vi "SRV_Watchdog Check Time.vi"(0 "System Config":T1={"SRV IP Address"="", "Video Stream Rate Period (ms)"=250, "Enable Diagnostic Log"=FALSE, "Watchdog 1 Config"={"Watchdog Name"="", "Watchdog Period (s)"=1.0, "Watchdog Command"={"I2C Address"=0, "Register"=0, "Value"=0, "Active"=FALSE}}, "Watchdog 2 Config"={"Watchdog Name"="", "Watchdog Period (s)"=1.0, "Watchdog Command"={"I2C Address"=0, "Register"=0, "Value"=0, "Active"=FALSE}}, "Sensor Window Filepath"=path ""} {"Watchdog 2 Config"."Watchdog Period (s)" format="%.3f"; "Watchdog 2 Config"."Watchdog Command"."Value" format="%02x"; "Watchdog 2 Config"."Watchdog Command"."Register" format="%02x"; "Watchdog 2 Config"."Watchdog Command"."I2C Address" format="%02x"; "Watchdog 1 Config"."Watchdog Period (s)" format="%.3f"; "Watchdog 1 Config"."Watchdog Command"."Value" format="%02x"; "Watchdog 1 Config"."Watchdog Command"."Register" format="%02x"; "Watchdog 1 Config"."Watchdog Command"."I2C Address" format="%02x"}, 7 "WD 1 Last Update":dbl, 9 "WD 2 Last Update":dbl, 11 "error in (no error)":errorcluster) -> (4 "System Config dup":T1={"SRV IP Address"="", "Video Stream Rate Period (ms)"=250, "Enable Diagnostic Log"=FALSE, "Watchdog 1 Config"={"Watchdog Name"="", "Watchdog Period (s)"=1.0, "Watchdog Command"={"I2C Address"=0, "Register"=0, "Value"=0, "Active"=FALSE}}, "Watchdog 2 Config"={"Watchdog Name"="", "Watchdog Period (s)"=1.0, "Watchdog Command"={"I2C Address"=0, "Register"=0, "Value"=0, "Active"=FALSE}}, "Sensor Window Filepath"=path ""} {"Watchdog 2 Config"."Watchdog Period (s)" format="%.3f"; "Watchdog 2 Config"."Watchdog Command"."Value" format="%02x"; "Watchdog 2 Config"."Watchdog Command"."Register" format="%02x"; "Watchdog 2 Config"."Watchdog Command"."I2C Address" format="%02x"; "Watchdog 1 Config"."Watchdog Period (s)" format="%.3f"; "Watchdog 1 Config"."Watchdog Command"."Value" format="%02x"; "Watchdog 1 Config"."Watchdog Command"."Register" format="%02x"; "Watchdog 1 Config"."Watchdog Command"."I2C Address" format="%02x"}, 6 "Current Time":dbl, 8 "Update WD 1?":bool, 10 "Update WD 2?":bool, 15 "error out":errorcluster)   [LabVIEW 2014]
uses:
  SubVIs/SysConfig/SRV_System Config.ctl
  SRV_Watchdog Config Cluster.ctl
  Motors/Motors Config/SRV_Motor Control Command Config.ctl
panel:
  # "I2C Address"
  # "Register"
  # "Value"
  # "Active"
  # "I2C Address"
  # "Register"
  # "Value"
  # "Active"
  # "I2C Address"
  # "Register"
  # "Value"
  # "Active"
  # "I2C Address"
  # "Register"
  # "Value"
  # "Active"
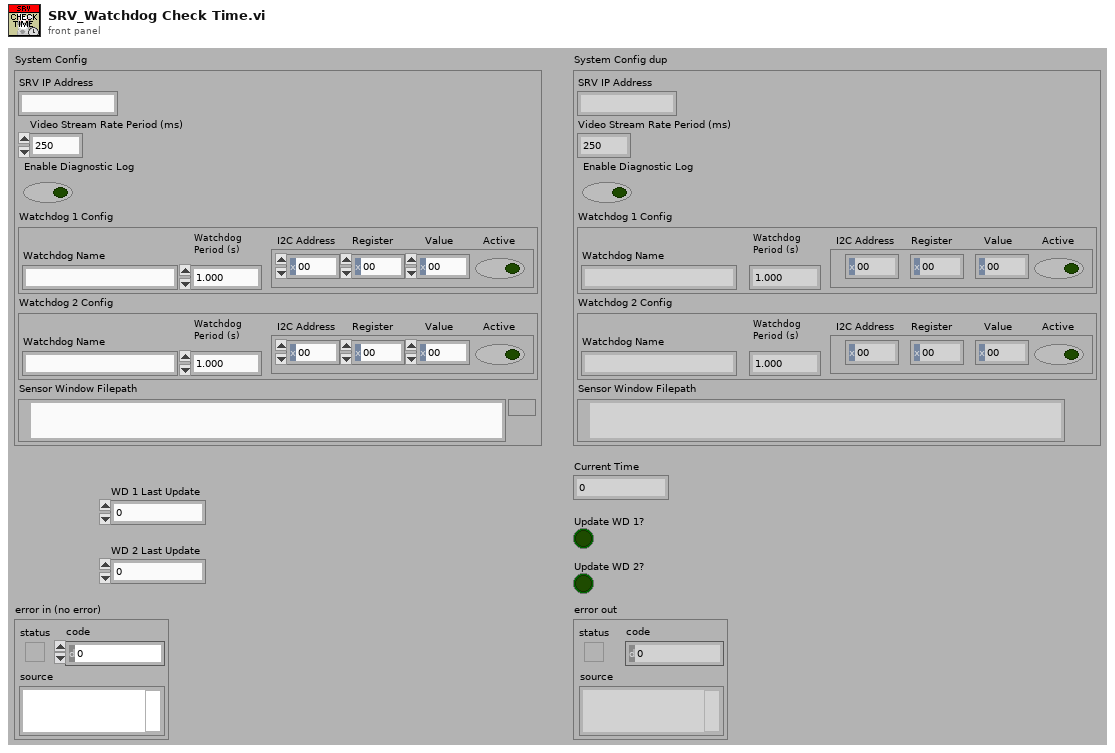
[diagram p1: front panel]
types:
  T1 = typedef "SRV_System Config.ctl" = cluster{"SRV IP Address":string, "Video Stream Rate Period (ms)":u32, "Enable Diagnostic Log":bool, "Watchdog 1 Config":T2, "Watchdog 2 Config":T2, "Sensor Window Filepath":path}
  T2 = typedef "SRV_Watchdog Config Cluster.ctl" = cluster{"Watchdog Name":string, "Watchdog Period (s)":dbl, "Watchdog Command":T3}
  T3 = typedef "SRV_Motor Control Command Config.ctl" = cluster{"I2C Address":u8, "Register":u8, "Value":u8, "Active":bool}
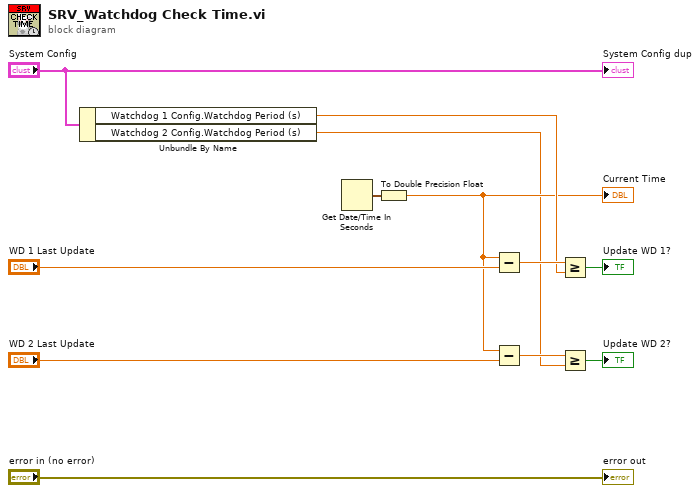
[diagram p0: block diagram]
diagram:
  n1 = Unbundle By Name("System Config") -> ("Watchdog 1 Config.Watchdog Period (s)"=w9:dbl, "Watchdog 2 Config.Watchdog Period (s)"=w3:dbl)
  n2 = Get Date/Time In Seconds() -> (seconds since 1Jan1904=w12:timestamp)
  n3 = To Double Precision Float(number=w12) -> (double precision float=w5:dbl)
  "Current Time" <- w5
  n4 = Subtract(x=w5, y="WD 1 Last Update") -> (x-y=w10:dbl)
  n5 = Subtract(x=w5, y="WD 2 Last Update") -> (x-y=w6:dbl)
  n6 = Greater Or Equal?(x=w10, y=w9) -> (x >= y?=→"Update WD 1?":bool)
  n7 = Greater Or Equal?(x=w6, y=w3) -> (x >= y?=→"Update WD 2?":bool)
  "error out" <- "error in (no error)"
  "System Config dup" <- "System Config"
